vi "TCP Write.vi"(8 "error in":errorcluster, 9 "timeout":i32, 10 "data":u8[](array[numeric]), 11 "connection ID":refnum<k5>) -> (0 "error out":errorcluster, 1 "timed out?":bool)   [LabVIEW 2021, in "TCP Shared Components.lvlib"]
doc: "This VI writes a set of data to a TCP connection and checks for errors. It is a wrapper for standard functionality."
uses:
  TCP Shared Components.lvlib
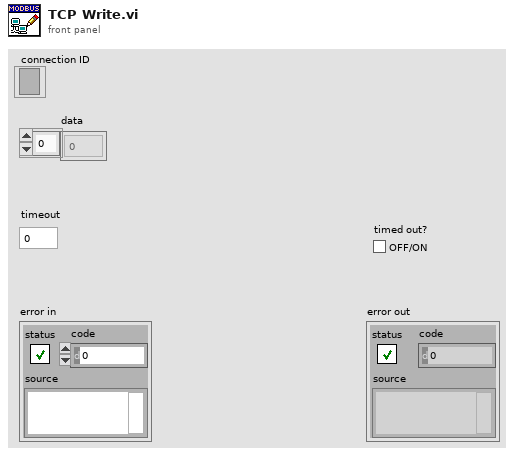
[diagram p1: front panel]
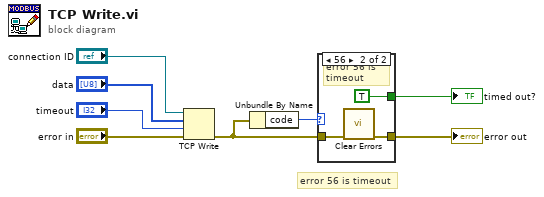
[diagram p0: block diagram]
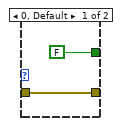
[diagram p2: hidden frame]
diagram:
  # "error 56 is timeout"
  n1 = TCP Write(connection ID="connection ID", data in="data", error in (no error)="error in", 9:"timeout") -> (error out=w2:errorcluster)  [unwired: 2 out]
  n2 = Unbundle By Name(w2) -> ("code"=w1:i32)
  n3 = case shown="56" w1 {
    tunnel: w2 -> [w10 w12]
    tunnel: [w10 w11] -> w5
    tunnel: [FALSE TRUE] -> w4
    frame 0, Default {
    }
    frame 56 {
      # "error 56 is timeout"
      n4 = call <vilib>:"Clear Errors.vi"("error in (no error)"=w12) -> ("error out"=w11:errorcluster)  [unwired: 5 in, 1 out]
    }
  }
  "error out" <- w5
  "timed out?" <- w4
